vi "Configure Power Measurement List Index.vi"(6 "Exp Nominal Power (-10)":dbl=-10.0, 7 "List Index (1)":i32=1, 8 "error in (no error)":errorcluster, 9 "Frequency (750MHz)":dbl=750000000.0 format="%#.9p", 10 "Instance (1)":i32=1 format="%.0g", 11 "VISA resource name":refnum<visa-resource-name>) -> (0 "error out":errorcluster, 3 "VISA resource name out":refnum<visa-resource-name>)   [LabVIEW 2015, in "Rohde&Schwarz CMXP GPRF.lvlib"]
doc: "Configures list of power measurement points.\n\nAttributes:\nRSCMXPGPRF_ATTR_SET_POWER_MEASUREMENT_LIST_STEP_FREQUENCY\nRSCMXPGPRF_ATTR_SET_POWER_MEASUREMENT_LIST_STEP_ENPOWER\n\nRemote-control commands:\nCONFigure:GPRF:MEAS<i>:POWer:LIST:FREQuency\nCONFigure:GPRF:MEAS<i>:POWer:LIST:ENPower"
uses:
  <instrlib>/Rohde&Schwarz CMXP GPRF/Rohde&Schwarz CMXP GPRF.lvlib
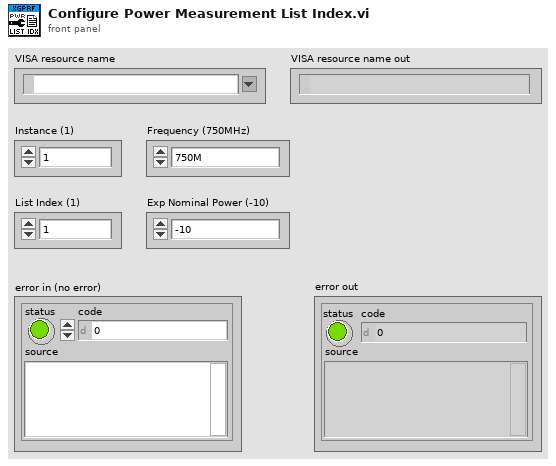
[diagram p1: front panel]
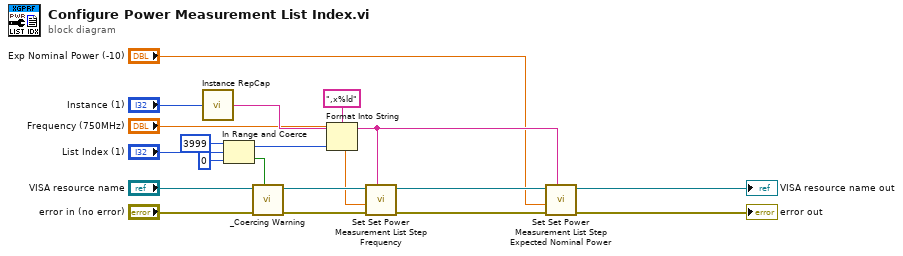
[diagram p0: block diagram]
diagram:
  n1 = call <instrlib>:"Instance RepCap.vi"("instance  in"="Instance (1)") -> ("instance out"=w19:string)
  n2 = In Range and Coerce(upper limit=3999, x="List Index (1)", lower limit=0) -> (coerced(x)=w3:i32, In Range?=w16:bool)
  n3 = call <instrlib>:"_Coercing Warning.vi"("In Range?"=w16, "error in (no error)"="error in (no error)", "VISA resource name"="VISA resource name") -> ("error out"=w14:errorcluster, "VISA resource name out"=w15:refnum<visa-resource-name>)  [unwired: 7 in]
  n4 = Format Into String(format string=",x%ld", initial string=w19, w3) -> (resulting string=w7:string)  [unwired: 1 in, 1 out]
  n5 = call "Set Set Power Measurement List Step Frequency"("Repeated Capabilities"=w7, "error in (no error)"=w14, "Set Power Measurement List Step Frequency (0.0)"="Frequency (750MHz)", "instrument handle"=w15) -> ("error out"=w8:errorcluster, "instrument handle out"=w9:refnum<visa-resource-name>)  [unwired: 6 in]
  n6 = call "Set Set Power Measurement List Step Expected Nominal Power"("Repeated Capabilities"=w7, "error in (no error)"=w8, "Set Power Measurement List Step Expected Nominal Power (0.0)"="Exp Nominal Power (-10)", "instrument handle"=w9) -> ("error out"=→"error out":errorcluster, "instrument handle out"=→"VISA resource name out":refnum<visa-resource-name>)  [unwired: 6 in]
